vi "Measurement Parser.vi"(7 "Waveform Graph":dynamicdata(graph), 8 "error in (no error)":errorcluster, 9 "Generic Card in":refnum<class "Generic Card.lvclass">, 10 "Data Array":dbl[](array[numeric]), 11 "AMS TCS3472 in":refnum<class "AMS TCS3472.lvclass">) -> (0 "error out":errorcluster, 3 "AMS TCS3472 out":refnum<class "AMS TCS3472.lvclass">)   [LabVIEW 2016, in "AMS TS3472 Light Sensor.lvlib" / "AMS TCS3472.lvclass"]
uses:
  AMS TCS3472.lvclass
  Generic Instrument/Generic Card/Generic Card.lvclass
  Abstract Sensor/Abstract Sensor.lvclass
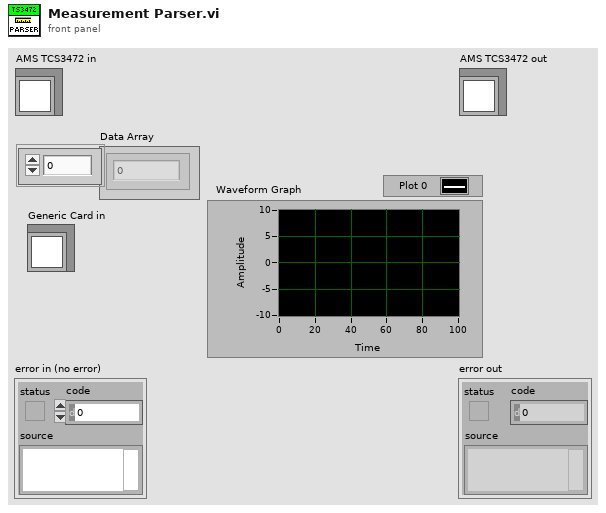
[diagram p1: front panel]
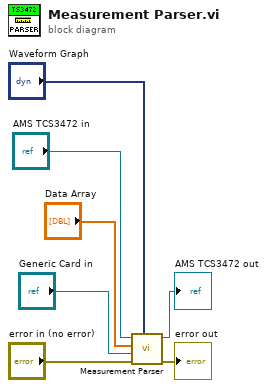
[diagram p0: block diagram]
diagram:
  n1 = call-parent "Measurement Parser.vi"("Waveform Graph"="Waveform Graph", "error in (no error)"="error in (no error)", "Generic Card in"="Generic Card in", "Data Array"="Data Array", "Abstract Sensor in"="AMS TCS3472 in") -> ("error out"=→"error out":errorcluster, "Abstract Sensor out"=→"AMS TCS3472 out":refnum<class "AMS TCS3472.lvclass">)  [unwired: 5 in]
